vi "DefaultConfigurationPath.vi"(8 "error in (no error)":errorcluster, 11 "SMO.UI.MAUI in":refnum<class "SMO.UI.MAUI.lvclass">) -> (0 "error out":errorcluster, 2 "Path":path, 3 "SMO.UI.MAUI out":refnum<class "SMO.UI.MAUI.lvclass">)   [LabVIEW 2020, in "SMO.UI.MAUI.lvclass"]
uses:
  SMO.UI.MAUI.lvclass
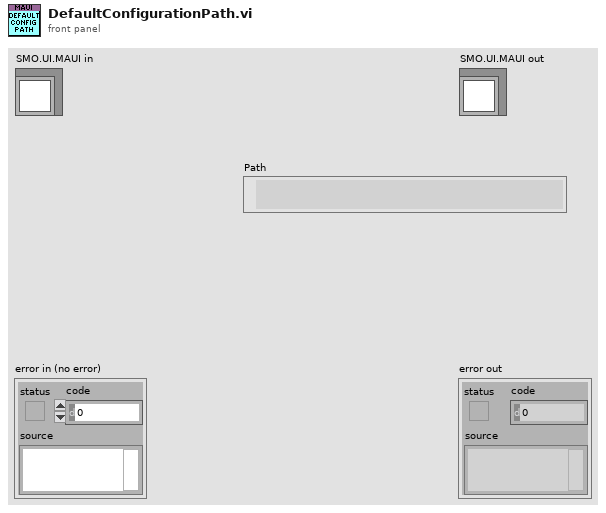
[diagram p1: front panel]
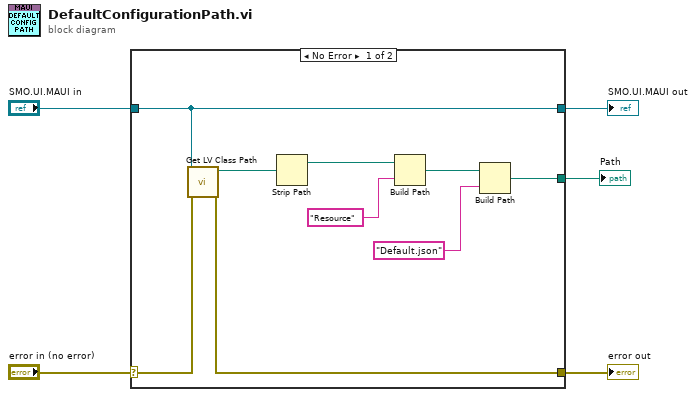
[diagram p0: block diagram]
diagram:
  n1 = case shown="No Error" "error in (no error)" {
    selector: "error in (no error)" -> [w8 w16]
    tunnel: [w7 w16] -> w4
    tunnel: [w14 w15] -> w2
    tunnel: "SMO.UI.MAUI in" -> [w14 w15]
    tunnel: [w6 _] -> w1
    frame No Error {
      n2 = call <vilib>:"Get LV Class Path.vi"("error in (no error)"=w8, "object"=w14) -> ("error out"=w7:errorcluster, "class path"=w13:path)  [unwired: 8 in]
      n3 = Strip Path(path=w13) -> (stripped path=w11:path)  [unwired: 1 out]
      n4 = Build Path(base path=w11, name or relative path="Resource") -> (appended path=w9:path)
      n5 = Build Path(base path=w9, name or relative path="Default.json") -> (appended path=w6:path)
    }
    frame Error {
    }
  }
  "error out" <- w4
  "SMO.UI.MAUI out" <- w2
  "Path" <- w1
